vi "OEE_SCREEN_2_build_stations_over_cycle_time_array.vi"(11 "SCREEN_1":T1) -> (3 "stations_over_cycle_time":i32[][](array[numeric]))   [LabVIEW 2019]
uses:
  <userlib>/_OpenG.lib/array/array.llb/Sort 2D Array (I32)__ogtk.vi
  SCREEN_1/typedef/SCREEN_1.ctl
panel:
  # "PERFORMANCE DATA OUTPUT BOARD #1"
  # "OP"
  # "Actual"
  # "Rejects"
  # "%FTTH"
  # "Pace"
  # "OP"
  # "Actual"
  # "Rejects"
  # "%FTTH"
  # "Pace"
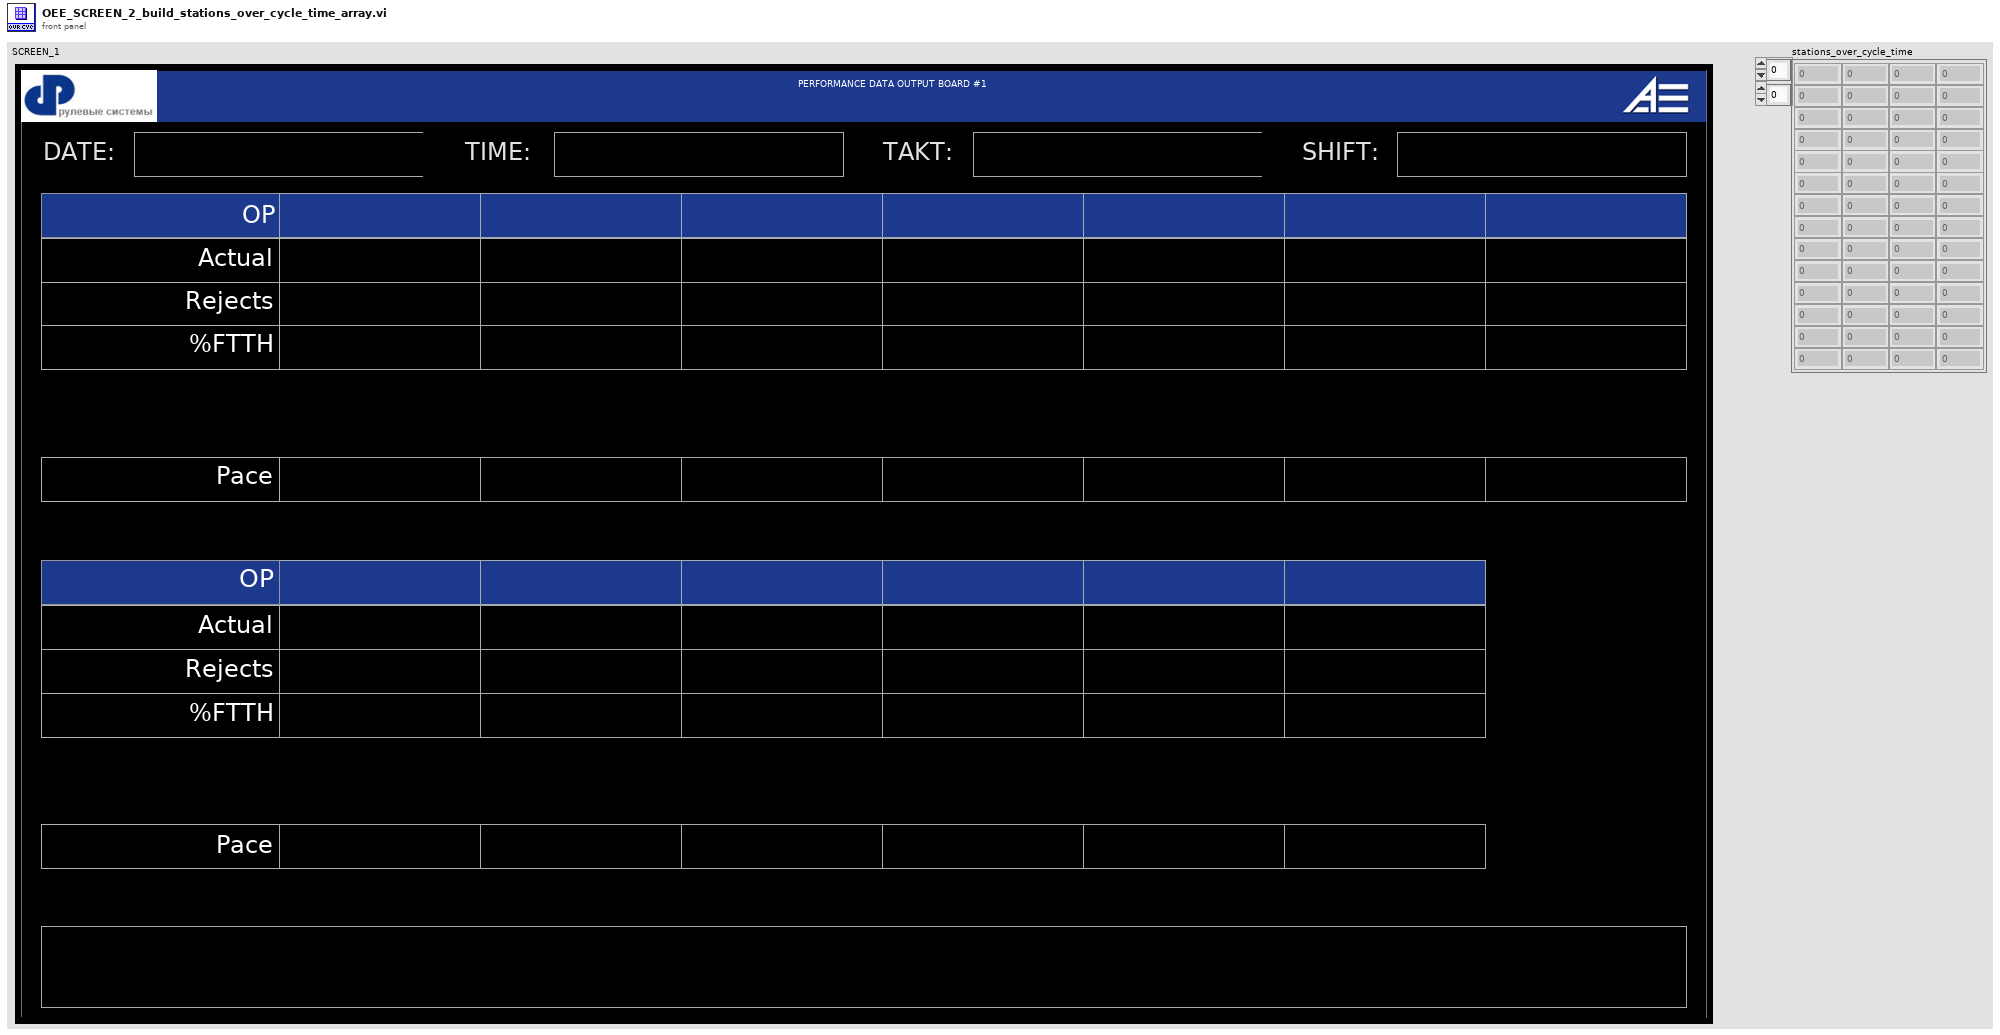
[diagram p1: front panel]
types:
  T1 = typedef "SCREEN_1.ctl" = cluster{"header_date":string, "header_time":string, "header_takt":string, "header_shift":string, "OP10_actual":string, "OP10_rejects":string, "OP10_quality_yeild":string, "OP10_pace":string, "OP20_actual":string, "OP20_rejects":string, "OP20_quality_yeild":string, "OP20_pace":string, "OP30_actual":string, "OP30_rejects":string, "OP30_quality_yeild":string, "OP30_pace":string, "OP40_actual":string, "OP40_rejects":string, "OP40_quality_yeild":string, "OP40_pace":string, "OP50_actual":string, "OP50_rejects":string, "OP50_quality_yeild":string, "OP50_pace":string, "OP60_actual":string, "OP60_rejects":string, "OP60_quality_yeild":string, "OP60_pace":string, "OP70_actual":string, "OP70_rejects":string, "OP70_quality_yeild":string, "OP70_pace":string, "OP80_actual":string, "OP80_rejects":string, "OP80_quality_yeild":string, "OP80_pace":string, "OP90_actual":string, "OP90_rejects":string, "OP90_quality_yeild":string, "OP90_pace":string, "OP100_actual":string, "OP100_rejects":string, "OP100_quality_yeild":string, "OP100_pace":string, "OP110_actual":string, "OP110_rejects":string, "OP110_quality_yeild":string, "OP110_pace":string, "OP120_actual":string, "OP120_rejects":string, "OP120_quality_yeild":string, "OP120_pace":string, "OP130_actual":string, "OP130_rejects":string, "OP130_quality_yeild":string, "OP130_pace":string, "OP10_header":string, "OP20_header":string, "OP30_header":string, "OP40_header":string, "OP50_header":string, "OP60_header":string, "OP70_header":string, "OP80_header":string, "OP90_header":string, "OP100_header":string, "OP110_header":string, "OP120_header":string, "OP130_header":string, "additional_info":string}
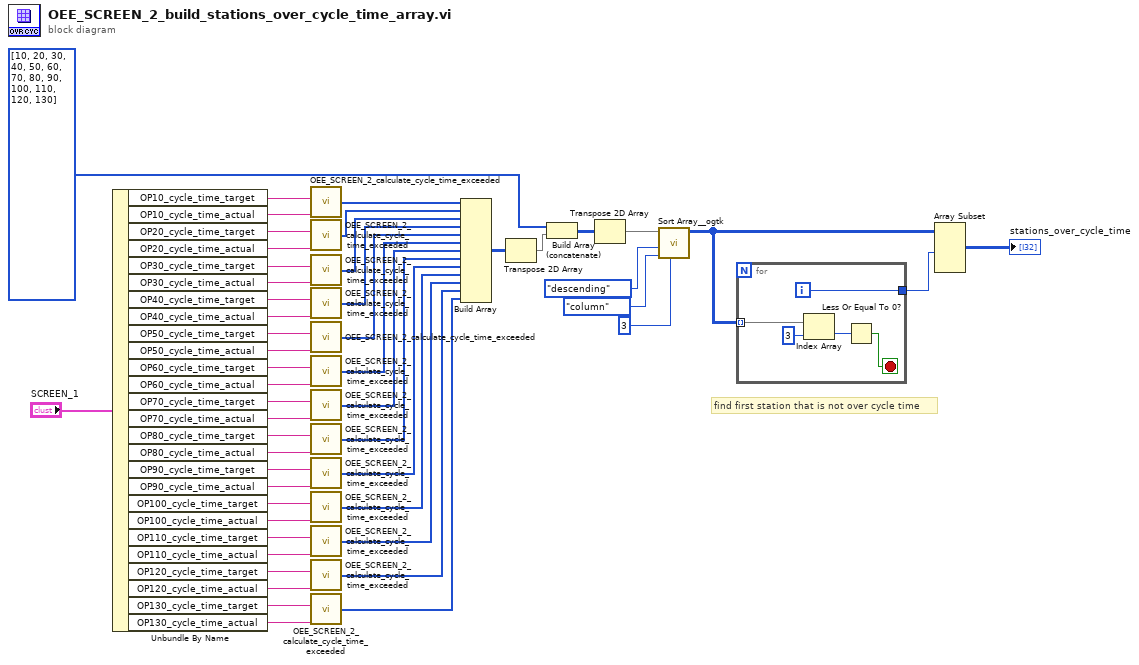
[diagram p0: block diagram]
diagram:
  # "find first station that is not over cycle time"
  n1 = Unbundle By Name("SCREEN_1") -> ("OP10_cycle_time_target"=w48:string, "OP10_cycle_time_actual"=w47:string, "OP20_cycle_time_target"=w45:string, "OP20_cycle_time_actual"=w40:string, "OP30_cycle_time_target"=w44:string, "OP30_cycle_time_actual"=w39:string, "OP40_cycle_time_target"=w43:string, "OP40_cycle_time_actual"=w2:string, "OP50_cycle_time_target"=w42:string, "OP50_cycle_time_actual"=w1:string, "OP60_cycle_time_target"=w41:string, "OP60_cycle_time_actual"=w38:string, "OP70_cycle_time_target"=w37:string, "OP70_cycle_time_actual"=w36:string, "OP80_cycle_time_target"=w35:string, "OP80_cycle_time_actual"=w34:string, "OP90_cycle_time_target"=w33:string, "OP90_cycle_time_actual"=w32:string, "OP100_cycle_time_target"=w31:string, "OP100_cycle_time_actual"=w30:string, "OP110_cycle_time_target"=w29:string, "OP110_cycle_time_actual"=w28:string, "OP120_cycle_time_target"=w27:string, "OP120_cycle_time_actual"=w26:string, "OP130_cycle_time_target"=w25:string, "OP130_cycle_time_actual"=w24:string)
  n2 = call "OEE_SCREEN_2_calculate_cycle_time_exceeded.vi"("cycle_time_actual"=w47, "cycle_time_target"=w48) -> ("target_actual_seconds_over"=w46:i32[])  [unwired: 2 in]
  n3 = call "OEE_SCREEN_2_calculate_cycle_time_exceeded.vi"("cycle_time_actual"=w40, "cycle_time_target"=w45) -> ("target_actual_seconds_over"=w23:i32[])  [unwired: 2 in]
  n4 = call "OEE_SCREEN_2_calculate_cycle_time_exceeded.vi"("cycle_time_actual"=w39, "cycle_time_target"=w44) -> ("target_actual_seconds_over"=w22:i32[])  [unwired: 2 in]
  n5 = call "OEE_SCREEN_2_calculate_cycle_time_exceeded.vi"("cycle_time_actual"=w2, "cycle_time_target"=w43) -> ("target_actual_seconds_over"=w21:i32[])  [unwired: 2 in]
  n6 = call "OEE_SCREEN_2_calculate_cycle_time_exceeded.vi"("cycle_time_actual"=w1, "cycle_time_target"=w42) -> ("target_actual_seconds_over"=w20:i32[])  [unwired: 2 in]
  n7 = call "OEE_SCREEN_2_calculate_cycle_time_exceeded.vi"("cycle_time_actual"=w38, "cycle_time_target"=w41) -> ("target_actual_seconds_over"=w19:i32[])  [unwired: 2 in]
  n8 = call "OEE_SCREEN_2_calculate_cycle_time_exceeded.vi"("cycle_time_actual"=w36, "cycle_time_target"=w37) -> ("target_actual_seconds_over"=w18:i32[])  [unwired: 2 in]
  n9 = call "OEE_SCREEN_2_calculate_cycle_time_exceeded.vi"("cycle_time_actual"=w34, "cycle_time_target"=w35) -> ("target_actual_seconds_over"=w17:i32[])  [unwired: 2 in]
  n10 = call "OEE_SCREEN_2_calculate_cycle_time_exceeded.vi"("cycle_time_actual"=w32, "cycle_time_target"=w33) -> ("target_actual_seconds_over"=w16:i32[])  [unwired: 2 in]
  n11 = call "OEE_SCREEN_2_calculate_cycle_time_exceeded.vi"("cycle_time_actual"=w30, "cycle_time_target"=w31) -> ("target_actual_seconds_over"=w15:i32[])  [unwired: 2 in]
  n12 = call "OEE_SCREEN_2_calculate_cycle_time_exceeded.vi"("cycle_time_actual"=w28, "cycle_time_target"=w29) -> ("target_actual_seconds_over"=w14:i32[])  [unwired: 2 in]
  n13 = call "OEE_SCREEN_2_calculate_cycle_time_exceeded.vi"("cycle_time_actual"=w26, "cycle_time_target"=w27) -> ("target_actual_seconds_over"=w13:i32[])  [unwired: 2 in]
  n14 = call "OEE_SCREEN_2_calculate_cycle_time_exceeded.vi"("cycle_time_actual"=w24, "cycle_time_target"=w25) -> ("target_actual_seconds_over"=w12:i32[])  [unwired: 2 in]
  n15 = Build Array(w46, w23, w22, w21, w20, w19, w18, w17, w16, w15, w14, w13, w12) -> (w11:i32[][])
  n16 = Transpose 2D Array(2D array=w11) -> (transposed array=w10:i32[][])
  n17 = Build Array (concatenate)(i32[] [10, 20, 30, 40, 50, 60, 70, 80, 90, 100, 110, 120, 130] ("appended array"), w10) -> (w50:i32[][])
  n18 = Transpose 2D Array(2D array=w50) -> (transposed array=w9:i32[][])
  n19 = call-poly <userlib>:"Sort Array__ogtk.vi"("Column/Row to Sort By"=u32 3, "Sort By in"=enum16{"row", "column"}."column", "Order"=enum16{"ascending", "descending"}."descending", "Array in"=w9) -> ("Sorted Array out"=w5:i32[][])  [unwired: 4 in, 3 out]
  n20 = for {
    tunnel: w5 -> [w56] mode=indexing
    tunnel: [w52] -> w3
    i -> [w52]
    stop <- w53 stop-if-true
    n21 = Index Array(array=w56, index=3) -> (element=w54:i32)
    n22 = Less Or Equal To 0?(x=w54) -> (x <= 0?=w53:bool)
  }
  n23 = Array Subset(array=w5, length (row)=w3) -> (→"stations_over_cycle_time":i32[][])  [unwired: 3 in]
